vi "grabber.vi"() -> ()   [LabVIEW 2010]
uses:
  <vilib>/Platform/TimedLoop/XDataNode/XDataNode.xnode
  <vilib>/Platform/TimedLoop/XDataNode/timing_clust.ctl
  <vilib>/Platform/TimedLoop/XDataNode/nitl_modes.ctl
  <vilib>/Platform/TimedLoop/XDataNode/wakeup.ctl
  <vilib>/dex/Flush And Wait Empty Condition.ctl
  <vilib>/rvi/interface/nirviMethod/nirviMethod.xnode
  <vilib>/rvi/interface/nirviReadWriteControl/nirviReadWriteControl.xnode
  <vilib>/rvi/interface/common/niFpgaNodeNameForErrorReporting.ctl
  <vilib>/rvi/errors/niLvFpgaWhatHappensToTopLevelVI.ctl
  scan_specification_cluster.ctl
  <vilib>/rvi/interface/nirviCloseFPGA/nirviCloseFPGA.xnode
  <vilib>/Utility/error.llb/Error Cluster From Error Code.vi
  <vilib>/rvi/errors/niLvFpgaAdjustHostInterfaceError.vi
  <vilib>/FPGAPlugInAG/Dynamic/niLvFpga_Close_Dynamic.vi
  <vilib>/Platform/TimedLoop/XDataNode/XDNodeRunTimeDep.lvlib
  NiFpgaLv.dll
panel:
  out "scan specification":T1
  out "read FIFO overflow duration [ms]":u32
  out "read pixels duration [ms]":u32
  out "stream pixels [ms]":u32
  in  "Close front-panel?":bool=TRUE
  out "initialised?":bool
  in  "stop":bool
  out "command lp err":errorcluster
  out "error out":errorcluster
  out "effective read-block size":u32
  in  "max read block size":u32=32000
  out "read loop ctr":i32
  out "pixels read from FPGA":u64
  out "elements in FPGA FIFO":u32
  out "last received command":string
  out "command loop finished":bool
  out "read loop finished":bool
  out "scanning?":bool
  out "FIFO overflow?":bool
  out "data read from FPGA FIFO":u32[](array[numeric])
  # "RealTime Grabber"
  # "Status"
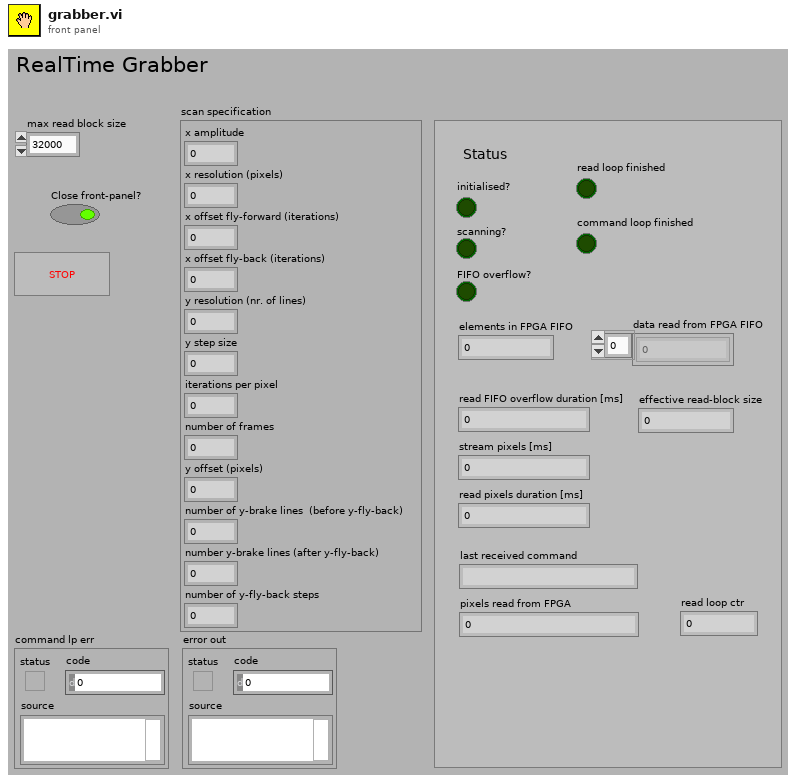
[diagram p1: front panel]
types:
  T1 = cluster{"x amplitude":u16, "x resolution (pixels)":u16, "x offset fly-forward (iterations)":u16, "x offset fly-back (iterations)":u16, "y resolution (nr. of lines)":u16, "y step size":u16, "iterations per pixel":u16, "number of frames":i32, "y offset (pixels)":u16, "number of y-brake lines  (before y-fly-back)":u16, "number y-brake lines (after y-fly-back)":u16, "number of y-fly-back steps":u16}
  T2 = typedef "network_streaming_queues_cluster.ctl" = cluster{"data writer endpoint":refnum<k21>, "command reader endpoint":refnum<k21>}
  T3 = typedef "XDNodeRunTimeDep.lvlib/timing_clust.ctl" = cluster{"Expected End [f-1]":u64, "Actual End [f-1]":u64, "Finished Late? [f-1]":bool, "Expected End [i-1]":u64, "Actual End [i-1]":u64, "Finished Late? [i-1]":bool, "Expected Start [i]":u64, "Actual Start [i]":u64, "Expected Start [f]":u64, "Actual Start [f]":u64, "Source Name":string, "Structure Name":string, "Period":i64, "Deadline":i64, "Offset":i64, "Start":i64, "Priority":i32, "Timeout":i32, "Mode":T4, "Wakeup Reason":T5, "Error":errorcluster, "Source Type":string, "Secondary Source Type":string, "Global End Time":u64, "Global Start Time":u64, "Frame Duration":u64, "Iteration Duration":u64, "Assigned CPU":i32, "I/O Scan Engine Mode":u32}
  T4 = typedef "XDNodeRunTimeDep.lvlib/nitl_modes.ctl" = enum32{"No Change", "Process missed periods, maintain original phase", "Discard missed periods, maintain original phase", "Process missed periods, ignore original phase", "Discard missed periods, ignore original phase"}
  T5 = typedef "XDNodeRunTimeDep.lvlib/wakeup.ctl" = enum32{"Normal", "Aborted", "Asynchronous wakeup", "Timing source error", "Timed loop error", "Timeout"}
  T6 = typedef "niFpgaNodeNameForErrorReporting.ctl" = enum16{"Open FPGA VI Reference", "Read/Write Control", "Invoke Method: Abort", "Invoke Method: Acknowledge IRQ", "Invoke Method: Download", "Invoke Method: FIFO.Configure", "Invoke Method: FIFO.Read", "Invoke Method: FIFO.Start", "Invoke Method: FIFO.Stop", "Invoke Method: FIFO.Write", "Invoke Method: Reset", "Invoke Method: Run", "Invoke Method: Wait on IRQ", "Close FPGA VI Reference"}
  T7 = typedef "niLvFpgaWhatHappensToTopLevelVI.ctl" = enum16{"top level VI scripted behind XNode", "top level VI inlined behind XNode"}
  T8 = typedef "Flush And Wait Empty Condition.ctl" = u8
  T9 = typedef "scan_specification_cluster.ctl" = cluster{"x amplitude":u16, "x resolution (pixels)":u16, "x offset fly-forward (iterations)":u16, "x offset fly-back (iterations)":u16, "y resolution (nr. of lines)":u16, "y step size":u16, "iterations per pixel":u16, "number of frames":i32, "y offset (pixels)":u16, "number of y-brake lines  (before y-fly-back)":u16, "number y-brake lines (after y-fly-back)":u16, "number of y-fly-back steps":u16}
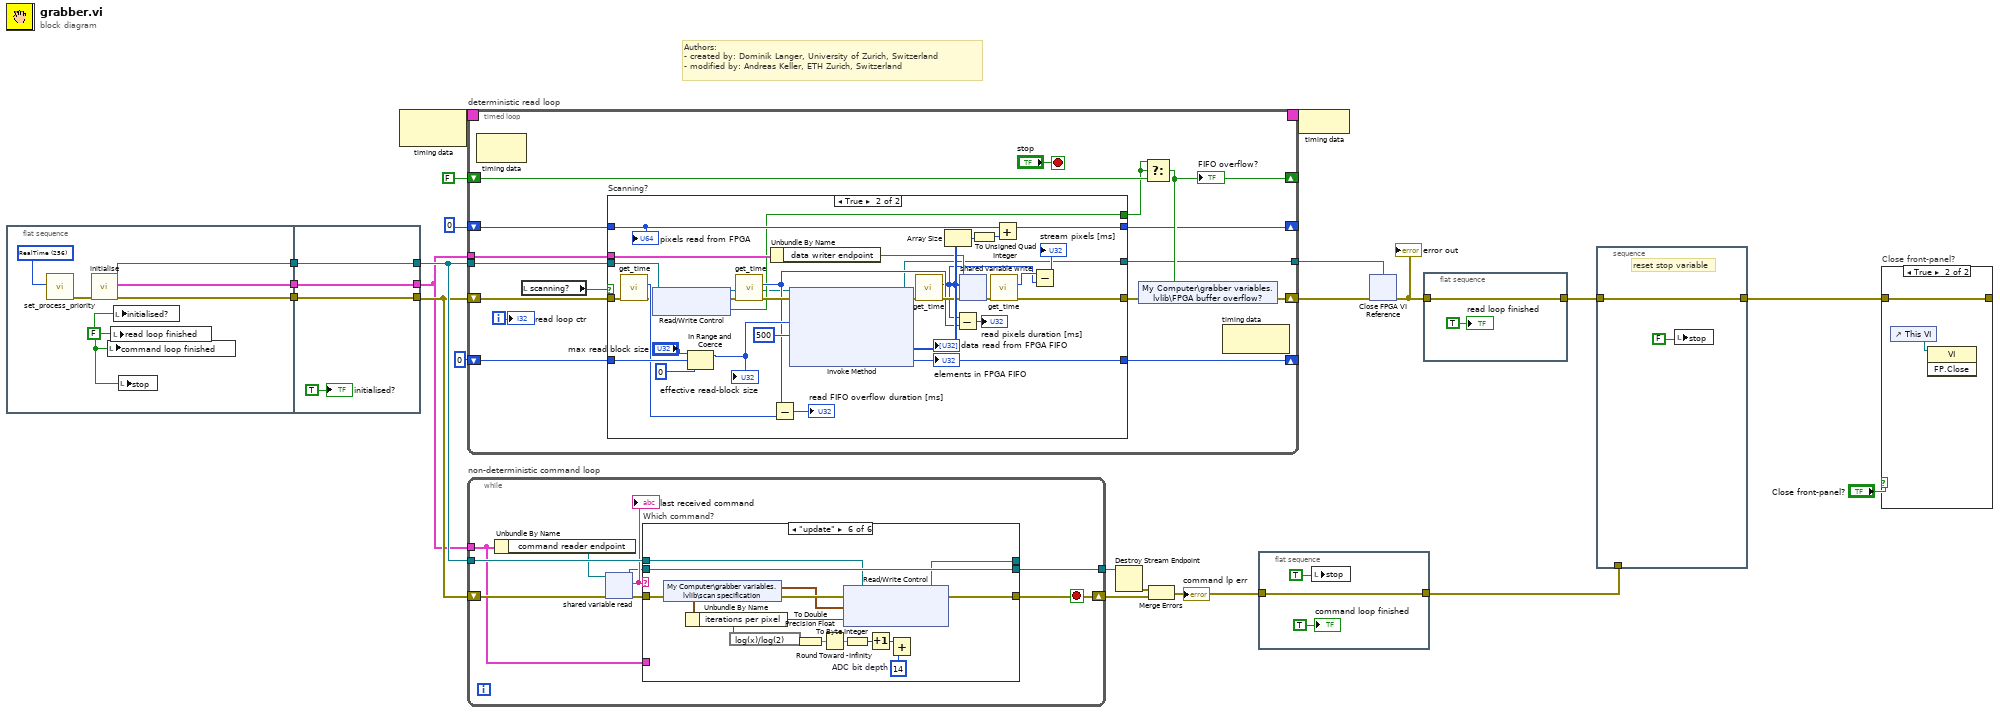
[diagram p0: block diagram]
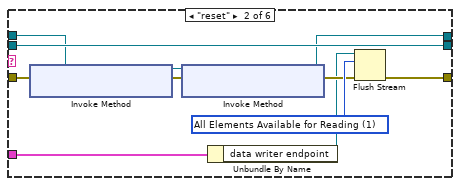
[diagram p4: hidden frame]
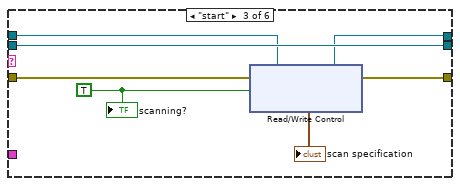
[diagram p5: hidden frame]
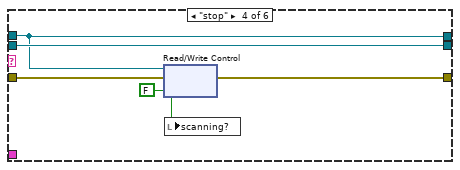
[diagram p6: hidden frame]
diagram:
  # "Authors: \n- created by: Dominik Langer, University of Zurich, Switzerland\n- modified by: Andreas Keller, ETH Zurich, Switzerland"
  n1 = flat-sequence {
    tunnel: [w26] -> w9
    tunnel: [w23] -> w8
    tunnel: [w24] -> w4
    tunnel: [w31] -> w20
    tunnel: [w32] -> w3
    tunnel: w9 -> [w32]
    tunnel: w8 -> [w31]
    tunnel: [w29] -> w2
    tunnel: w4 -> [w29]
    frame #0 {
      w25 = FALSE ("read loop finished")
      w28 = 256 items=["Normal"=32, "Idle"=64, "High"=128, "RealTime"=256, "BelowNormal"=16384, "AboveNormal"=32768] ("PriorityClass")
      n2 = call "set_process_priority.vi"("PriorityClass"=w28) -> ("error out"=w27:errorcluster)  [unwired: 10 in]
      n3 = call "initialise.vi"("error in (no error)"=w27) -> ("error out"=w26:errorcluster, "network streaming queues"=w24:T2, "FPGA VI Reference Out"=w23:refnum<k20>)  [unwired: 8 in]
      n4 = local write "command loop finished"(w25) -> ()
      n5 = local write "read loop finished"(w25) -> ()
      n6 = local write "initialised?"(w25) -> ()
      n7 = local write "stop"(w25) -> ()
    }
    frame #1 {
      "initialised?" <- TRUE ("initialised?")
    }
  }
  n8 = node-c288 ("Input Node")() -> (w22:T3)  [unwired: 1 in]
  n9 = timed-loop "deterministic read loop" {
    timing: w22 -> [_]
    timing-out: [_] -> w21
    shift-right: [w40] -> w14
    shift-left: w3 -> [w38]
    tunnel: w20 -> [w33]
    shift-right: [w47] -> _
    shift-left: FALSE ("FIFO overflow") -> [w48]
    shift-right: [w44] -> _
    shift-left: u64 0 -> [w46]
    tunnel: [w42] -> w13
    shift-right: [w36] -> _
    shift-left: u32 0 ("Elements Remaining") -> [w35]
    tunnel: w2 -> [w34]
    i -> [w45]
    stop <- "stop" stop-if-true
    n10 = node-c288 ("Output Node")() -> ()  [unwired: 1 in, 1 out]
    n11 = local read "scanning?"() -> (w37:bool)
    n12 = case "Scanning?" shown="True" w37 {
      tunnel: w38 -> [w52 w63]
      tunnel: [w52 w67] -> w41
      tunnel: w33 -> [w51 w55]
      tunnel: [w51 w53] -> w42
      tunnel: w46 -> [_ w76]
      tunnel: [_ w83] -> w44
      tunnel: [_ w57] -> w43
      tunnel: [_ w78] -> w36
      tunnel: w35 -> [_ w77]
      tunnel: w34 -> [_ w73]
      frame False {
      }
      frame True {
        n13 = call "get_time.vi"("error in (no error)"=w63) -> ("error out"=w58:errorcluster, "millisecond timer value"=w62:u32)  [unwired: 9 in]
        n14 = xnode "Read/Write Control"("FPGA VI Reference In"=w55, "error in"=w58) -> ("FPGA VI Reference Out"=w54:refnum<k20>, "error out"=w56:errorcluster, "FIFO overflow"=w57:bool)
        n15 = In Range and Coerce(upper limit="max read block size", x=w77, lower limit=u32 0) -> (coerced(x)=w75:u32)  [unwired: 1 out]
        "effective read-block size" <- w75
        n16 = call "get_time.vi"("error in (no error)"=w56) -> ("error out"=w65:errorcluster, "millisecond timer value"=w60:u32)  [unwired: 9 in]
        n17 = Unbundle By Name(w73) -> ("data writer endpoint"=w72:refnum<k21>)
        n18 = Subtract(x=w60, y=w62) -> (x-y=→"read FIFO overflow duration [ms]":u32)
        n19 = xnode "Invoke Method"("FPGA VI Reference In"=w54, "error in"=w65, "Number of Elements"=w75, "Timeout (ms)"=500) -> ("FPGA VI Reference Out"=w53:refnum<k20>, "error out"=w70:errorcluster, "Data"=w74:u32[], "Elements Remaining"=w78:u32)
        "data read from FPGA FIFO" <- w74
        "elements in FPGA FIFO" <- w78
        n20 = call "get_time.vi"("error in (no error)"=w70) -> ("error out"=w69:errorcluster, "millisecond timer value"=w59:u32)  [unwired: 9 in]
        n21 = Array Size(array=w74) -> (size(s)=w84:i32)
        n22 = Subtract(x=w59, y=w60) -> (x-y=→"read pixels duration [ms]":u32)
        n23 = shared-variable-write(w72, w69, w74) -> (w68:errorcluster)  [unwired: 1 in, 2 out]
        n24 = To Unsigned Quad Integer(1:w84) -> (0:w82:u64)
        n25 = call "get_time.vi"("error in (no error)"=w68) -> ("error out"=w67:errorcluster, "millisecond timer value"=w66:u32)  [unwired: 9 in]
        n26 = Add(x=w76, y=w82) -> (x+y=w83:u64)
        n27 = Subtract(x=w66, y=w59) -> (x-y=→"stream pixels [ms]":u32)
        "pixels read from FPGA" <- w76
      }
    }
    n28 = Select(t=w43, s=w43, f=w48) -> (s? t:f=w47:bool)
    "FIFO overflow?" <- w47
    n29 = shared-variable "My Computer\\grabber variables.lvlib\\FPGA buffer overflow?"(w47, error in=w41) -> (error out=w40:errorcluster)
    n30 = node-c288 ("Input Node")() -> ()  [unwired: 1 in, 1 out]
    "read loop ctr" <- w45
  }
  n31 = while "non-deterministic command loop" {
    shift-right: [w203] -> w12
    shift-left: w3 -> [w209]
    tunnel: w20 -> [w208]
    tunnel: [w204] -> w19
    tunnel: w2 -> [w201]
    stop <- w203 stop-if-true
    n32 = Unbundle By Name(w201) -> ("command reader endpoint"=w202:refnum<k21>)
    n33 = shared-variable-read(w202, w209) -> (w205:refnum<k21>, w207:errorcluster, w206:string)  [unwired: 1 in, 1 out]
    "last received command" <- w206
    n34 = case "Which command?" shown="\"update\"" w206 {
      tunnel: w208 -> [w210 w221 w272 w350 w392 w399]
      tunnel: w207 -> [w212 w223 w270 w349 w391 w407]
      tunnel: [w212 w215 w274 w347 w391 w397] -> w203
      tunnel: w205 -> [w211 w222 w273 w351 w393 w400]
      tunnel: [w211 w222 w273 w351 w393 w400] -> w204
      tunnel: [w210 w220 w271 w350 w392 w398] -> _
      tunnel: w201 -> [_ w214 _ _ _ _]
      frame "NULL", Default {
      }
      frame "reset" {
        w217 = T8 1 items=["All Elements Read From Stream", "All Elements Available for Reading"] ("wait condition")
        n35 = xnode "Invoke Method"("FPGA VI Reference In"=w221, "error in"=w223) -> ("FPGA VI Reference Out"=w218:refnum<k20>, "error out"=w219:errorcluster)
        n36 = xnode "Invoke Method"("FPGA VI Reference In"=w218, "error in"=w219) -> ("FPGA VI Reference Out"=w220:refnum<k20>, "error out"=w216:errorcluster)
        n37 = Unbundle By Name(w214) -> ("data writer endpoint"=w213:refnum<k21>)
        n38 = Flush Stream(8:w216, 10:w217, 11:w213) -> (0:w215:errorcluster)  [unwired: 1 in, 2 out]
      }
      frame "start" {
        w269 = TRUE ("scan")
        n39 = xnode "Read/Write Control"("FPGA VI Reference In"=w272, "error in"=w270, "scan"=w269) -> ("FPGA VI Reference Out"=w271:refnum<k20>, "error out"=w274:errorcluster, "scan specification"=→"scan specification":T1)
        "scanning?" <- w269
      }
      frame "stop" {
        w348 = FALSE ("scan")
        n40 = xnode "Read/Write Control"("FPGA VI Reference In"=w350, "error in"=w349, "scan"=w348) -> ("error out"=w347:errorcluster)  [unwired: 1 out]
        n41 = local write "scanning?"(w348) -> ()
      }
      frame "terminate" {
      }
      frame "update" {
        w403 = i8 14  # ADC bit depth
        n42 = shared-variable "My Computer\\grabber variables.lvlib\\scan specification"(error in=w407) -> (w395:T9, error out=w396:errorcluster)
        n43 = Unbundle By Name(w395) -> ("iterations per pixel"=w394:u16)
        n44 = expression code="log(x)/log(2)"(w394) -> (w401:u16)
        n45 = To Double Precision Float(number=w401) -> (double precision float=w404:dbl)
        n46 = Round Toward -Infinity(1:w404) -> (0:w402:dbl)
        n47 = xnode "Read/Write Control"("FPGA VI Reference In"=w399, "error in"=w396, "scan specification"=w395, "maximum bit depth"=w394) -> ("FPGA VI Reference Out"=w398:refnum<k20>, "error out"=w397:errorcluster)
        n48 = To Byte Integer(number=w402) -> (8bit integer=w405:i8)
        n49 = Increment(x=w405) -> (x+1=w406:i8)
        n50 = Add(x=w406, y=w403) -> ()  [unwired: 1 out]
      }
    }
  }
  n51 = Destroy Stream Endpoint(11:w19) -> (0:w11:errorcluster)  [unwired: 1 in]
  n52 = Merge Errors(w11, w12) -> (w10:errorcluster)
  "command lp err" <- w10
  n53 = flat-sequence {
    tunnel: w10 -> [w473]
    tunnel: [w473] -> w18
    frame #0 {
      n54 = local write "stop"(TRUE ("stop - RT")) -> ()
      "command loop finished" <- TRUE ("command loop finished")
    }
  }
  n55 = node-c288 ("Output Node")(w21) -> ()
  n56 = xnode "Close FPGA VI Reference"("FPGA VI Reference In"=w13, "error in"=w14) -> ("error out"=w1:errorcluster)
  "error out" <- w1
  n57 = flat-sequence {
    tunnel: w1 -> [w477]
    tunnel: [w477] -> w17
    frame #0 {
      "read loop finished" <- TRUE ("read loop finished")
    }
  }
  n58 = stacked-sequence {
    tunnel: w18 -> [_]
    tunnel: w17 -> [w478]
    tunnel: [w478] -> w6
    frame #0 {
      # "reset stop variable"
      n59 = local write "stop"(FALSE) -> ()
    }
  }
  n60 = case "Close front-panel?" shown="True" "Close front-panel?" {
    tunnel: [w480 w481] -> _
    tunnel: w6 -> [w480 w481]
    frame False {
    }
    frame True {
      n61 = control-ref of="This VI"() -> (w482:refnum<vi>)
      n62 = invoke class="VI" method="FP.Close"(reference=w482) -> ()  [unwired: 2 in, 3 out]
    }
  }
